vi "Pre Launch Init.vi"(11 "Nested in":refnum<class "GUI Generador.lvclass">) -> (0 "error out":errorcluster, 3 "Nested out":refnum<class "GUI Generador.lvclass">)   [LabVIEW 2020, in "GUI Generador.lvlib" / "GUI Generador.lvclass"]
doc: "(<B>Filename</B>: Actor Framework.lvlib:Actor.lvclass:Pre Launch Init.vi)\n\nDefines behavior that occurs after the Launch Nested Actor method is invoked but before the actor's Actor Core method begins running.\n\nBy default, this method does nothing. A descendant class may override it to define behavior."
uses:
  GUI Generador.lvclass
  GUI Generador.lvclass/GUI Generador.ctl
  <vilib>/ActorFramework/Actor/Actor.lvclass
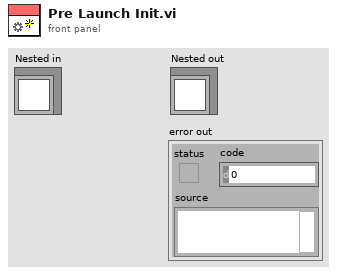
[diagram p1: front panel]
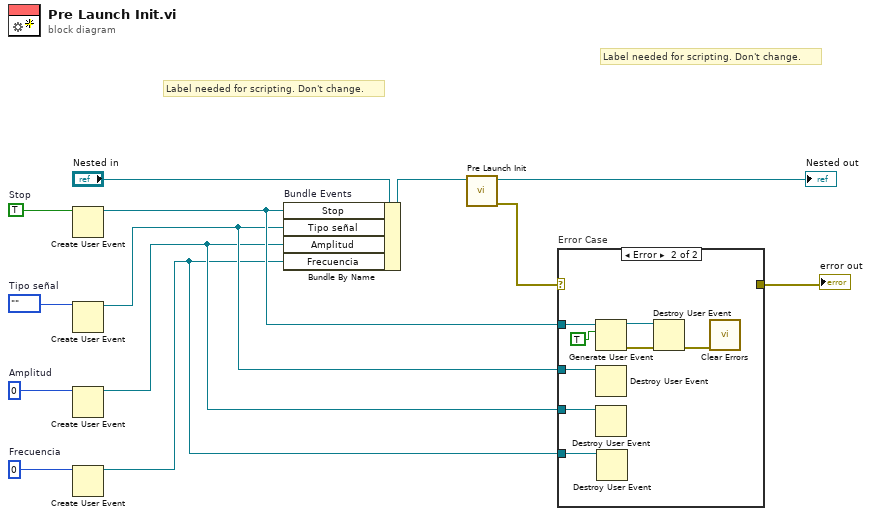
[diagram p0: block diagram]
diagram:
  w5 = TRUE  # Stop
  w7 = 0  # Frecuencia
  w8 = 0  # Amplitud
  w9 = enum16{""}.""  # Tipo señal
  # "Label needed for scripting. Don't change."
  # "Label needed for scripting. Don't change."
  n1 = Create User Event(user event datatype=w5) -> (user event=w4:refnum<user-event>)  [unwired: 1 in, 1 out]
  n2 = Create User Event(user event datatype=w9) -> (user event=w3:refnum<user-event>)  [unwired: 1 in, 1 out]
  n3 = Create User Event(user event datatype=w8) -> (user event=w2:refnum<user-event>)  [unwired: 1 in, 1 out]
  n4 = Create User Event(user event datatype=w7) -> (user event=w1:refnum<user-event>)  [unwired: 1 in, 1 out]
  n5 = Bundle By Name "Bundle Events"(cluster="Nested in", "Stop"=w4, "Tipo señal"=w3, "Amplitud"=w2, "Frecuencia"=w1) -> (w11:refnum<class "GUI Generador.lvclass">)
  n6 = call-parent "Pre Launch Init.vi"("Actor in"=w11) -> ("error out"=w10:errorcluster, "Actor out"=→"Nested out":refnum<class "GUI Generador.lvclass">)  [unwired: 9 in]
  n7 = case "Error Case" shown="Error" w10 {
    selector: w10 -> [w14 _]
    tunnel: [w14 _] -> w12
    tunnel: w4 -> [_ w22]
    tunnel: w3 -> [_ w20]
    tunnel: w2 -> [_ w19]
    tunnel: w1 -> [_ w18]
    frame No Error {
    }
    frame Error {
      n8 = Generate User Event(user event=w22, event data cluster=TRUE ("event data")) -> (user event out=w17:refnum<user-event>, error out=w21:errorcluster)  [unwired: 2 in]
      n9 = Destroy User Event(user event=w20) -> ()  [unwired: 1 in, 1 out]
      n10 = Destroy User Event(user event=w19) -> ()  [unwired: 1 in, 1 out]
      n11 = Destroy User Event(user event=w18) -> ()  [unwired: 1 in, 1 out]
      n12 = Destroy User Event(user event=w17, error in=w21) -> (error out=w15:errorcluster)
      n13 = call <vilib>:"Clear Errors.vi"("error in (no error)"=w15) -> ()  [unwired: 5 in, 2 out]
    }
  }
  "error out" <- w12
